vi "x_O.vi"(2 "Tic Tac Toe":i8[][](array[numeric])) -> (6 "GrafikRing":i32[][](array[numeric]), 10 "Game":i32[][](array[numeric]))   [LabVIEW 2017]
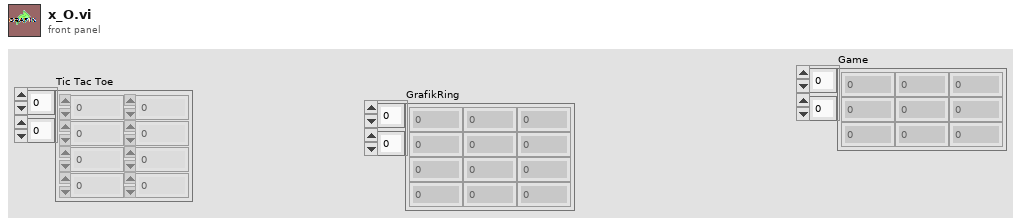
[diagram p1: front panel]
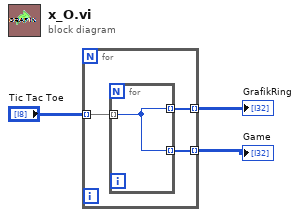
[diagram p0: block diagram]
diagram:
  n1 = for {
    tunnel: "Tic Tac Toe" -> [w5] mode=indexing
    tunnel: [w6] -> w2 mode=indexing
    tunnel: [w4] -> w1 mode=indexing
    n2 = for {
      tunnel: [w7] -> w6 mode=indexing
      tunnel: w5 -> [w7] mode=indexing
      tunnel: [w7] -> w4 mode=indexing
    }
  }
  "GrafikRing" <- w2
  "Game" <- w1
